vi "mod.vi"(8 "Divide":i16, 11 "Value In":i16) -> (0 "Ceil":i16, 3 "Value out":i16)   [LabVIEW 2023]
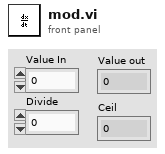
[diagram p1: front panel]
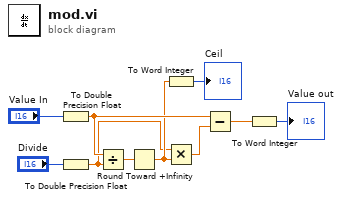
[diagram p0: block diagram]
diagram:
  n1 = To Double Precision Float(number="Value In") -> (double precision float=w7:dbl)
  n2 = To Double Precision Float(number="Divide") -> (double precision float=w1:dbl)
  n3 = Divide(x=w7, y=w1) -> (x/y=w10:dbl)
  n4 = Round Toward +Infinity(x=w10) -> (ceil(x): smallest int >= x=w4:dbl)
  n5 = To Word Integer(number=w4) -> (16bit integer=→"Ceil":i16)
  n6 = Multiply(x=w1, y=w4) -> (x*y=w9:dbl)
  n7 = Subtract(x=w7, y=w9) -> (x-y=w6:dbl)
  n8 = To Word Integer(number=w6) -> (16bit integer=→"Value out":i16)
